vi "Test Indexing.vi"(8 "error in (no error)":errorcluster) -> (0 "error out":errorcluster)   [LabVIEW 2020]
uses:
  b06a4517-5669-43fd-b225-d6aa28537e4c.vi
  6e754613-e0ce-43fb-8ab0-88c5f5e7dd3c.vi
  f8314fe3-53d2-45e6-92eb-a9411662c67d.vi
  d83e61e9-b517-4a5e-86ec-54f9338e1657.vi
  8e2a0650-45f6-4a14-b352-b1eeae9abe12.vi
  e6ed8b94-1348-4b4a-b4cb-83684bf9a3c3.vi
  b06a4517-5669-43fd-b225-d6aa28537e4c.vi/e73b2968-3a52-4c27-a773-88fb5d420c14.vi
  6e754613-e0ce-43fb-8ab0-88c5f5e7dd3c.vi/5edf5e06-e093-4a0f-aa29-e2cbb43d817c.vi
  6e754613-e0ce-43fb-8ab0-88c5f5e7dd3c.vi/74f13dcf-f2a8-47e7-a307-5a2d66421bf6.vi
  <vilib>/Utility/error.llb/Error Cluster From Error Code.vi
  <vilib>/addons/_JKI Toolkits/Caraya/classes/Assert/Assert Equal Value and Type_Variant.vi
  <vilib>/addons/_JKI Toolkits/Caraya/classes/Assert/Assert Error.vi
  <vilib>/addons/_JKI Toolkits/Caraya/classes/Assert/Assert False.vi
  <vilib>/addons/_JKI Toolkits/Caraya/classes/Test/Test.lvclass
  <vilib>/addons/_JKI Toolkits/Caraya/classes/Assert/Assert.lvclass
  Source/VIM Tools.lvlib
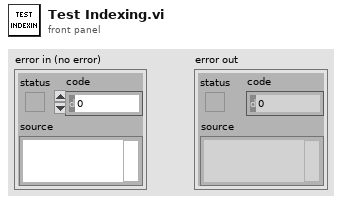
[diagram p1: front panel]
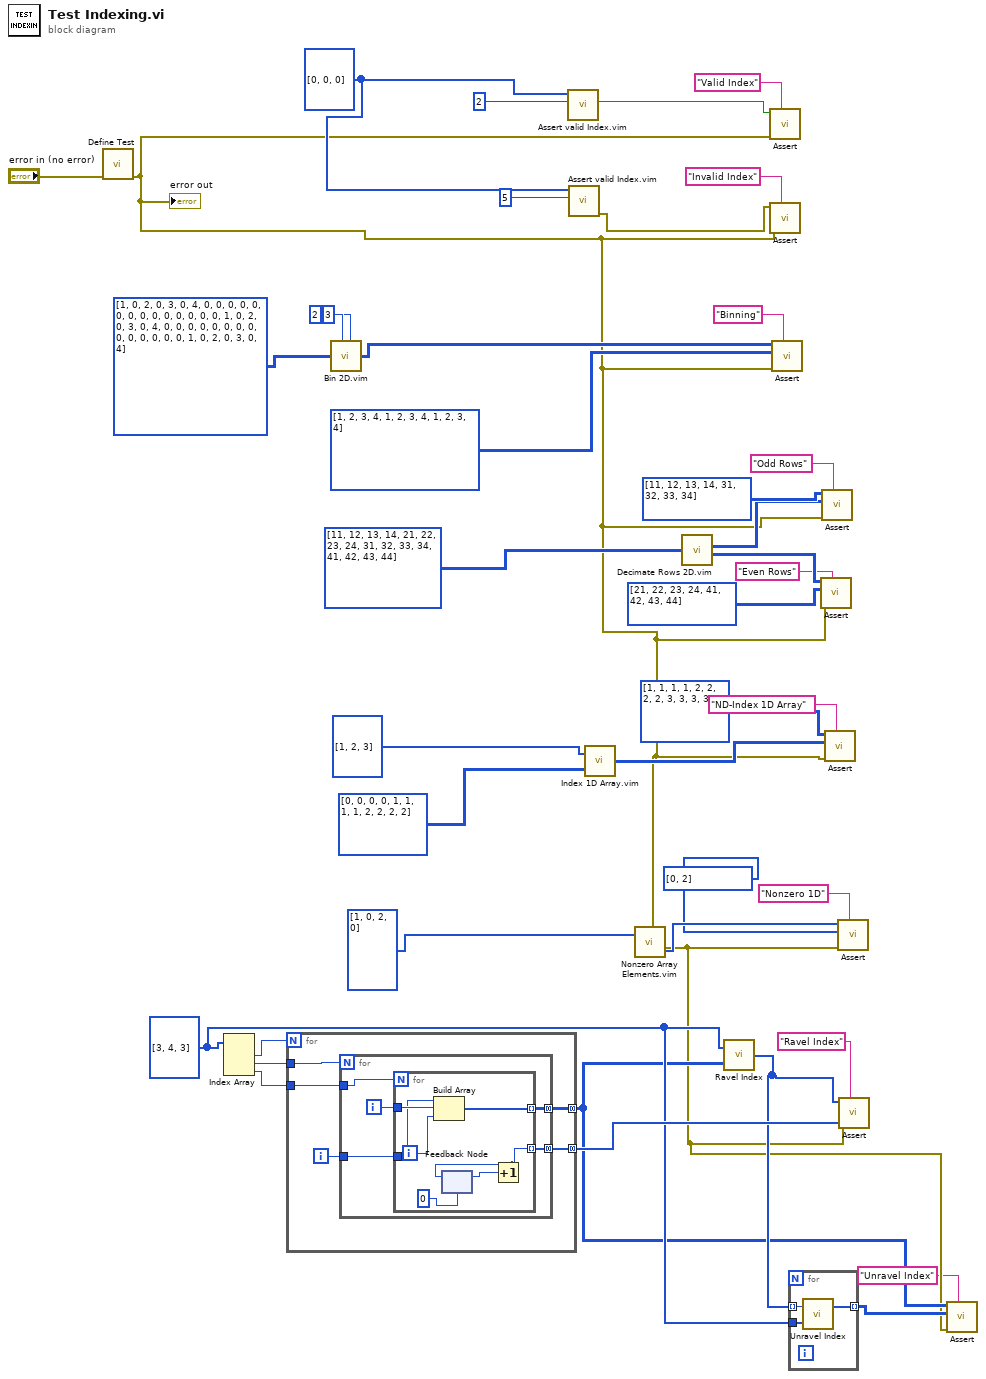
[diagram p0: block diagram]
diagram:
  w7 = i32[] [3, 4, 3]
  w36 = i32[] [0, 0, 0]
  n1 = call <vilib>:"Define Test.vi"("error in (no error)"="error in (no error)") -> ("error out"=w3:errorcluster)  [unwired: 10 in]
  "error out" <- w3
  n2 = Index Array(array=w7) -> (element #1=w10:i32, element #2=w9:i32, element #3=w8:i32)  [unwired: 3 in]
  n3 = for {
    N: w10 -> [_]
    tunnel: [w45] -> w4 mode=concatenating
    tunnel: [w44] -> w12 mode=concatenating
    tunnel: w9 -> [w43]
    tunnel: w8 -> [w42]
    i -> [w46]
    n4 = for {
      N: w43 -> [_]
      tunnel: w46 -> [w50]
      tunnel: [w49] -> w45 mode=concatenating
      tunnel: [w48] -> w44 mode=concatenating
      tunnel: w42 -> [w47]
      i -> [w51]
      n5 = for {
        N: w47 -> [_]
        tunnel: w51 -> [w58]
        tunnel: w50 -> [w57]
        tunnel: [w56] -> w49 mode=indexing
        tunnel: [w55] -> w48 mode=indexing
        i -> [w52]
        n6 = Build Array(w57, w58, w52) -> (w56:i32[])
        n7 = feedback #1(0) -> (w55:i32)
        n8 = Increment(x=w55) -> (x+1=w53:i32)
        n9 = feedback-in #1(w53) -> ()
      }
    }
  }
  n10 = call "Bin 2D.vim"("Bin Dim 1"=2, "Array"=i32[][] [[1, 0, 2, 0, 3, 0, 4], [0, 0, 0, 0, 0, 0, 0], [0, 0, 0, 0, 0, 0, 0], [1, 0, 2, 0, 3, 0, 4], [0, 0, 0, 0, 0, 0, 0], [0, 0, 0, 0, 0, 0, 0], [1, 0, 2, 0, 3, 0, 4]], "Bin Dim 2"=3) -> ("Binned Array"=w31:i32[][])  [unwired: 6 in]
  n11 = call "Assert valid Index.vim"("index"=2, "Array"=w36) -> ("Index Invalid?"=w40:bool)  [unwired: 8 in, 1 out]
  n12 = call "Assert valid Index.vim"("index"=5, "Array"=w36) -> ("error out"=w35:errorcluster)  [unwired: 8 in, 1 out]
  n13 = call "Index 1D Array.vim"("Indices"=i32[][] [[0, 0, 0, 0], [1, 1, 1, 1], [2, 2, 2, 2]], "Array"=i32[] [1, 2, 3]) -> ("Indexed Elements"=w18:i32[][])
  n14 = call "Nonzero Array Elements.vim"("Array"=i32[] [1, 0, 2, 0]) -> ("Flat Index"=w15:i32[])  [unwired: 1 in, 1 out]
  n15 = call "Decimate Rows 2D.vim"("2D Array In"=i32[][] [[11, 12, 13, 14], [21, 22, 23, 24], [31, 32, 33, 34], [41, 42, 43, 44]] ("Binned Array")) -> ("Odd Rows Out"=w24:i32[][], "Even Rows Out"=w27:i32[][])  [unwired: 6 in]
  n16 = call "Ravel Index.vi"("ND Indices"=w4, "Array Shape"=w7) -> ("Flat Indices"=w6:i32[])  [unwired: 1 in]
  n17 = call-poly <vilib>:"Assert.vi"("Label"="Valid Index", "error in (no error)"=w3, "False?"=w40) -> ()  [unwired: 8 in, 1 out]
  n18 = call-poly <vilib>:"Assert.vi"("Label"="Invalid Index", "error in (no error)"=w3, "Error?"=w35) -> ()  [unwired: 8 in, 1 out]
  n19 = call-poly <vilib>:"Assert.vi"("Label"="Binning", "error in (no error)"=w3, "Y"=i32[][] [[1, 2, 3, 4], [1, 2, 3, 4], [1, 2, 3, 4]] ("Binned Array"), "X"=w31) -> ()  [unwired: 7 in, 1 out]
  n20 = for {
    tunnel: w7 -> [w61]
    tunnel: w6 -> [w60] mode=indexing
    tunnel: [w59] -> w5 mode=indexing
    n21 = call "Unravel Index.vi"("shape"=w61, "Flat Index"=w60) -> ("ND Index"=w59:i32[])  [unwired: 1 out]
  }
  n22 = call-poly <vilib>:"Assert.vi"("Label"="Even Rows", "error in (no error)"=w3, "Y"=i32[][] [[21, 22, 23, 24], [41, 42, 43, 44]] ("Even Rows Out"), "X"=w27) -> ()  [unwired: 7 in, 1 out]
  n23 = call-poly <vilib>:"Assert.vi"("Label"="Odd Rows", "error in (no error)"=w3, "Y"=w24, "X"=i32[][] [[11, 12, 13, 14], [31, 32, 33, 34]] ("Even Rows Out")) -> ()  [unwired: 7 in, 1 out]
  n24 = call-poly <vilib>:"Assert.vi"("Label"="ND-Index 1D Array", "error in (no error)"=w3, "Y"=w18, "X"=i32[][] [[1, 1, 1, 1], [2, 2, 2, 2], [3, 3, 3, 3]] ("Indexed Elements")) -> ()  [unwired: 7 in, 1 out]
  n25 = call-poly <vilib>:"Assert.vi"("Label"="Nonzero 1D", "error in (no error)"=w3, "Y"=i32[] [0, 2] ("Flat Index"), "X"=w15) -> ()  [unwired: 7 in, 1 out]
  n26 = call-poly <vilib>:"Assert.vi"("Label"="Ravel Index", "error in (no error)"=w3, "Y"=w12, "X"=w6) -> ()  [unwired: 7 in, 1 out]
  n27 = call-poly <vilib>:"Assert.vi"("Label"="Unravel Index", "error in (no error)"=w3, "Y"=w5, "X"=w4) -> ()  [unwired: 7 in, 1 out]
